vi "Write to FPGA.vi"(7 "Queue in":refnum<queue>, 8 "error in (no error)":errorcluster, 11 "FPGA VI Reference In":refnum<k20>) -> (0 "error out":errorcluster, 3 "FPGA VI Reference Out":refnum<k20>)   [LabVIEW 2015]
uses:
  <vilib>/Utility/error.llb/Error Cluster From Error Code.vi
  <vilib>/rvi/errors/niLvFpgaAdjustHostInterfaceError.vi
  <vilib>/rvi/interface/nirviReadWriteControl/nirviReadWriteControl.xnode
  NiFpgaLv.dll
  <vilib>/rvi/interface/Simulation/niFpgaSimulationCallBeginRW.vi
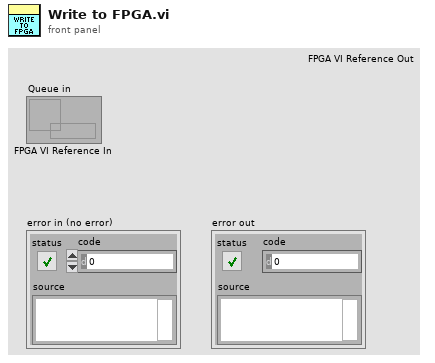
[diagram p1: front panel]
types:
  T1 = cluster{"Gas Value":dbl, "Knob Value":i16, "DIR":bool, "Stepper ON":bool, "DoorA":bool, "DoorB":bool, "wiper":bool, "Lights 1":bool, "Lights 2":bool, "Turn Signal":i8, "BREAK":bool, "Start Engine":bool, "Undder LIghts":bool}
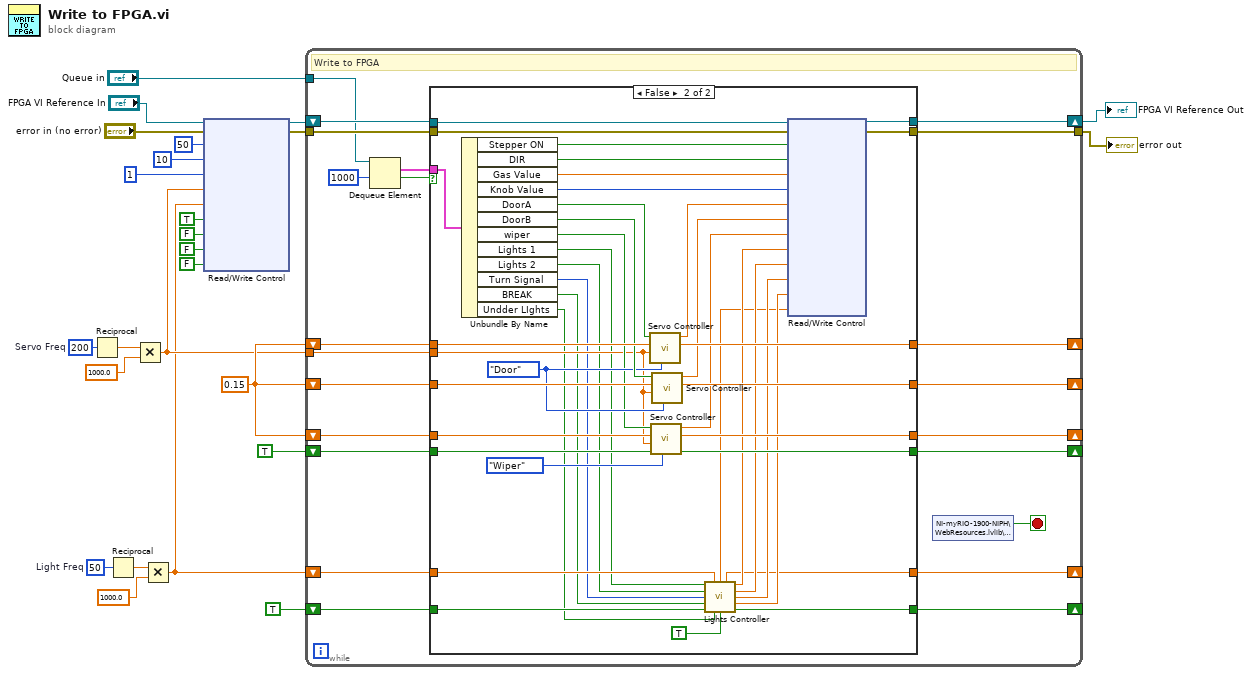
[diagram p0: block diagram]
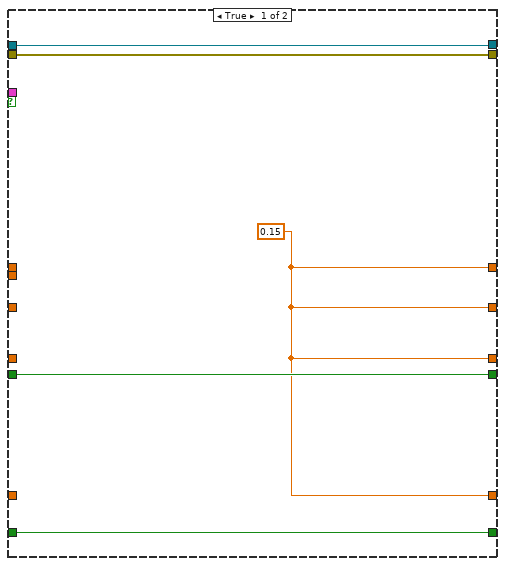
[diagram p2: hidden frame]
diagram:
  w24 = u32 50  # Light Freq
  w19 = 0.15 ("y")
  w15 = u32 200  # Servo Freq
  n1 = Reciprocal(x=w15) -> (1/x=w16:dbl)
  n2 = Reciprocal(x=w24) -> (1/x=w23:dbl)
  n3 = Multiply(x=w16, y=1000.0) -> (x*y=w18:dbl)
  n4 = Multiply(x=w23, y=1000.0) -> (x*y=w1:dbl)
  n5 = xnode "Read/Write Control"("FPGA VI Reference In"="FPGA VI Reference In", "error in"="error in (no error)", "Count(mSec)"=u32 50, "Period"=u32 10, "Pulse Width"=u32 1, "Servo Period"=w18, "Lights Period"=w1, "LED0"=TRUE, "LED1"=FALSE, "LED2"=FALSE, "LED3"=FALSE) -> ("FPGA VI Reference Out"=w12:refnum<k20>, "error out"=w13:errorcluster)
  n6 = while {
    tunnel: w13 -> [w47]
    tunnel: [w45] -> w14
    tunnel: "Queue in" -> [w43]
    shift-right: [w46] -> w4
    shift-left: w12 -> [w44]
    shift-right: [w41] -> _
    shift-left: w19 -> [w42]
    tunnel: w18 -> [w40]
    shift-right: [w39] -> _
    shift-left: w19 -> [w38]
    shift-right: [w37] -> _
    shift-left: w19 -> [w36]
    shift-right: [w35] -> _
    shift-left: TRUE ("Wiper Flag Shift Reg") -> [w34]
    shift-right: [w32] -> _
    shift-left: TRUE ("Wiper Flag Shift Reg") -> [w33]
    shift-right: [w30] -> _
    shift-left: w1 -> [w31]
    stop <- w27 stop-if-true
    # "Write to FPGA"
    n7 = Dequeue Element(queue=w43, timeout in ms (-1)=1000) -> (element=w29:T1, timed out?=w26:bool)  [unwired: 1 in, 2 out]
    n8 = case shown="False" w26 {
      tunnel: w47 -> [w51 w93]
      tunnel: [w52 w92] -> w46
      tunnel: [w51 w91] -> w45
      tunnel: w44 -> [w52 w90]
      tunnel: w29 -> [_ w68]
      tunnel: w42 -> [_ w82]
      tunnel: [w49 w84] -> w41
      tunnel: w40 -> [_ w71]
      tunnel: [w49 w80] -> w39
      tunnel: w38 -> [_ w79]
      tunnel: [w49 w73] -> w37
      tunnel: w36 -> [_ w72]
      tunnel: [w50 w70] -> w35
      tunnel: w34 -> [w50 w69]
      tunnel: w33 -> [w48 w67]
      tunnel: [w48 w66] -> w32
      tunnel: w31 -> [_ w65]
      tunnel: [w49 w60] -> w30
      frame True {
        w49 = 0.15 ("y")
      }
      frame False {
        w77 = enum16{"Door", "Wiper"}."Door" ("Enum")
        n9 = Unbundle By Name(w68) -> ("Stepper ON"=w89:bool, "DIR"=w88:bool, "Gas Value"=w86:dbl, "Knob Value"=w87:i16, "DoorA"=w85:bool, "DoorB"=w78:bool, "wiper"=w75:bool, "Lights 1"=w59:bool, "Lights 2"=w58:bool, "Turn Signal"=w57:i8, "BREAK"=w56:bool, "Undder LIghts"=w54:bool)
        n10 = call "Servo Controller.vi"("Enum"=w77, "Servo Period"=w71, "Duty min"=w82, "Door"=w85) -> ("Shift Reg"=w84:dbl, "Door Duty"=w83:dbl)  [unwired: 5 in, 1 out]
        n11 = call "Servo Controller.vi"("Enum"=enum16{"Door", "Wiper"}."Wiper", "Wiper Flag"=w69, "Servo Period"=w71, "Duty min"=w72, "Door"=w75) -> ("Wiper Flag Shift Reg"=w70:bool, "Shift Reg"=w73:dbl, "Door Duty"=w74:dbl)  [unwired: 4 in]
        n12 = call "Servo Controller.vi"("Enum"=w77, "Servo Period"=w71, "Duty min"=w79, "Door"=w78) -> ("Shift Reg"=w80:dbl, "Door Duty"=w81:dbl)  [unwired: 5 in, 1 out]
        n13 = call "Lights Controller.vi"("Lights 1"=w59, "Light Period"=w65, "Lights 2"=w58, "Turn Signal"=w57, "Break"=w56, "Lights Flag"=w67, "Under Lights"=w54, "Start Engine"=TRUE) -> ("Blue Duty"=w53:dbl, "Light Period Out"=w60:dbl, "Red  Duty"=w64:dbl, "White Duty"=w63:dbl, "Orange L Duty"=w61:dbl, "Orange R Duty"=w62:dbl, "Lights Flag Out"=w66:bool)  [unwired: 1 in]
        n14 = xnode "Read/Write Control"("FPGA VI Reference In"=w90, "error in"=w93, "Stepper ON"=w89, "DIRECTION"=w88, "GAS"=w86, "Steering"=w87, "DoorA Duty"=w83, "DoorB Duty"=w81, "Wiper Duty"=w74, "R duty"=w64, "W duty"=w63, "OL Duty"=w61, "OR Duty"=w62, "B Duty"=w53) -> ("FPGA VI Reference Out"=w92:refnum<k20>, "error out"=w91:errorcluster)
      }
    }
    n15 = shared-variable "NI-myRIO-1900-NIPH\\WebResources.lvlib\\Engine"() -> (w27:bool)  [unwired: 1 in, 1 out]
  }
  "error out" <- w14
  "FPGA VI Reference Out" <- w4
